vi "Check_Folder Exist.vi"(10 "Folder Name":string, 11 "Root Folder":path) -> (3 "Output Path":path)   [LabVIEW 2012]
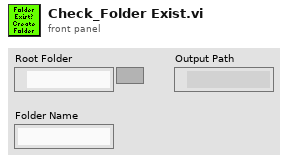
[diagram p1: front panel]
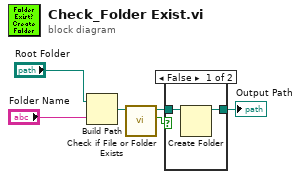
[diagram p0: block diagram]
diagram:
  n1 = Build Path(base path="Root Folder", name or relative path="Folder Name") -> (appended path=w4:path)
  n2 = call <vilib>:"Check if File or Folder Exists.vi"("path"=w4) -> ("file or folder exists?"=w2:bool, "dup path"=w3:path)  [unwired: 8 in, 1 out]
  n3 = case shown="False" w2 {
    tunnel: w3 -> [w8 w9]
    tunnel: [w7 w9] -> w5
    frame False {
      n4 = Create Folder(path (use dialog)=w8) -> (created path=w7:path)  [unwired: 2 in, 2 out]
    }
    frame True {
    }
  }
  "Output Path" <- w5
